vi "Sub_Preprocessing_LEMP_Initialize.vi"(1 "Stiff":T2, 2 "Mass":T2) -> (0 "LEMP":T1)   [LabVIEW 2021]
uses:
  <vilib>/Analysis/Matrix/Datatypes/RealMatrix.ctl
  <vilib>/Analysis/Matrix/Numeric/Conversions/Matrix To Array - RM.vi
  <vilib>/Analysis/Matrix/Numeric/Conversions/Matrix To Array - CM.vi
  <vilib>/Analysis/Matrix/NI_Matrix.lvlib
panel:
  # "Input"
  # "Output"
  # "This VI acquires the required input cluster for the Sub_online_LEMP_Update.vi, this VI calls on SciPy.linalg.eigh() due to issues with the standard \"General Eigenvalues and Eigenvectors.vi\" outputting inappropriately scaled eigenvectors for the LEMP. Additionally the Bitedness of this installation of LabVIEW does not match with Python so direct python calls were similarly unavailable. The workaround involved a saving the matrices in a text format command line calling the SciPy eigh function saving that output as a text file, then load the output file in to memory (See Sub_Python_cmd_eigh.vi, getEigenCommandPrompt.py , mass.lvm, stiff.lvm,eigenvalues.txt, eigenvectors.txt).\n\n              - Alexander Vereen AFRL Summer scholars 2022"
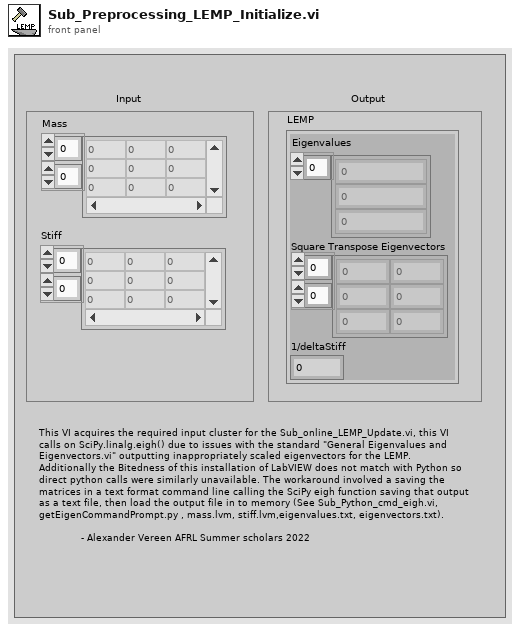
[diagram p1: front panel]
types:
  T1 = cluster{"Eigenvalues":dbl[], "Square Transpose Eigenvectors":dbl[][], "1/deltaStiff":dbl}
  T2 = typedef "NI_Matrix.lvlib/RealMatrix.ctl" = dbl[][]
  T3 = typedef "NI_Matrix.lvlib/ComplexMatrix.ctl" = cdb[][]
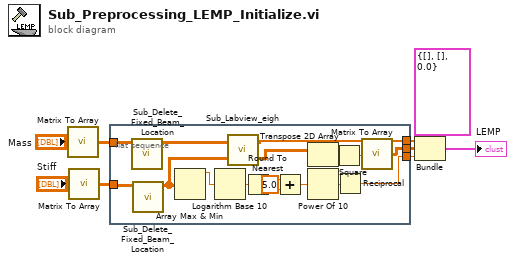
[diagram p0: block diagram]
diagram:
  n1 = call-poly <vilib>:"Matrix To Array.vi"("Real Matrix"="Mass") -> ("Real 2D Array"=w1:dbl[][])
  n2 = call-poly <vilib>:"Matrix To Array.vi"("Real Matrix"="Stiff") -> ("Real 2D Array"=w8:dbl[][])
  n3 = flat-sequence {
    tunnel: [w10] -> w5
    tunnel: [w22] -> w4
    tunnel: [w23] -> w3
    tunnel: w1 -> [w21]
    tunnel: w8 -> [w20]
    frame #0 {
      n4 = call "Sub_Delete_Fixed_Beam_Location.vi"("Pre-BC Matrix"=w21) -> ("Post-BC Matrix"=w13:dbl[][])  [unwired: 10 in]
      n5 = call "Sub_Delete_Fixed_Beam_Location.vi"("Pre-BC Matrix"=w20) -> ("Post-BC Matrix"=w12:dbl[][])  [unwired: 10 in]
      n6 = Array Max & Min(array=w12) -> (max value=w14:dbl)  [unwired: 3 out]
      n7 = Logarithm Base 10(1:w14) -> (0:w17:dbl)
      n8 = call "Sub_Labview_eigh.vi"("Stiffness"=w12, "Mass"=w13) -> ("Eigenvectors"=w11:T3, "Eigenvalues"=w10:dbl[])
      n9 = Round To Nearest(number=w17) -> (nearest integer value=w18:dbl)
      n10 = Add(x=w18, y=5.0) -> (x+y=w19:dbl)
      n11 = Transpose 2D Array(2D array=w11) -> (transposed array=w25:T3)
      n12 = Power Of 10(x=w19) -> (10^x=w15:dbl)
      n13 = Square(x=w25) -> (x^2=w24:T3)
      n14 = Reciprocal(x=w15) -> (1/x=w23:dbl)
      n15 = call-poly <vilib>:"Matrix To Array.vi"("Complex Matrix"=w24) -> ("Complex 2D Array"=w22:cdb[][])
    }
  }
  n16 = Bundle(cluster=T1 {"Eigenvalues"=[], "Square Transpose Eigenvectors"=[], "1/deltaStiff"=0.0} ("LEMP"), "Eigenvalues"=w5, "Square Transpose Eigenvectors"=w4, "1/deltaStiff"=w3) -> (→"LEMP":T1)
